vi "PutPlayerTrajectoryOnBoard.vi"(8 "error in (no error)":errorcluster, 9 "PlayerID":string="p1", 10 "PlayerTrajectory":T1[](array[typedef]), 11 "Board in":T4[][](array[typedef])) -> (0 "error out":errorcluster, 3 "Board out":T4[][](array[typedef]))   [LabVIEW 2015, in "TronviewPresentation.lvlib" / "BoardDisplay.lvclass"]
uses:
  BoardDisplay.lvclass
  TrajectoryBoardField.ctl
  TrajectoryFieldType.ctl
  TronVIEWBotAPI/MovementDirection.ctl
  PlayerTrajectory.ctl
  TronviewGame/Board/Position.ctl
  TronVIEWBotAPI/TronVIEWBotAPI.lvlib
  TronviewGame/Board/Board.lvclass
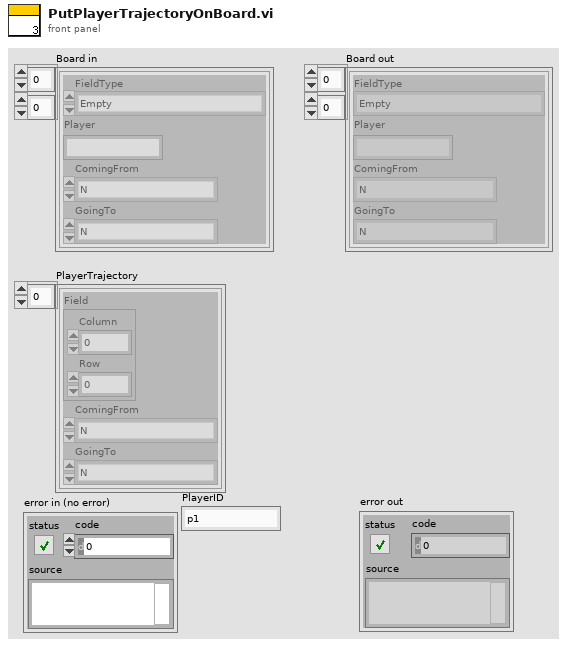
[diagram p1: front panel]
types:
  T1 = typedef "TronviewPresentation.lvlib/BoardDisplay.lvclass/PlayerTrajectory.ctl" = cluster{"Field":T2, "ComingFrom":T3, "GoingTo":T3}
  T2 = typedef "TronviewGame.lvlib/Board.lvclass/Position.ctl" = cluster{"Column":i32, "Row":i32}
  T3 = typedef "TronVIEWBotAPI.lvlib/MovementDirection.ctl" = enum16{"N", "S", "W", "E"}
  T4 = typedef "TronviewPresentation.lvlib/BoardDisplay.lvclass/TrajectoryBoardField.ctl" = cluster{"FieldType":T5, "Player":string, "ComingFrom":T3, "GoingTo":T3}
  T5 = typedef "TronviewPresentation.lvlib/BoardDisplay.lvclass/TrajectoryFieldType.ctl" = enum16{"Empty", "Initial", "PlayerWall", "PlayerPosition"}
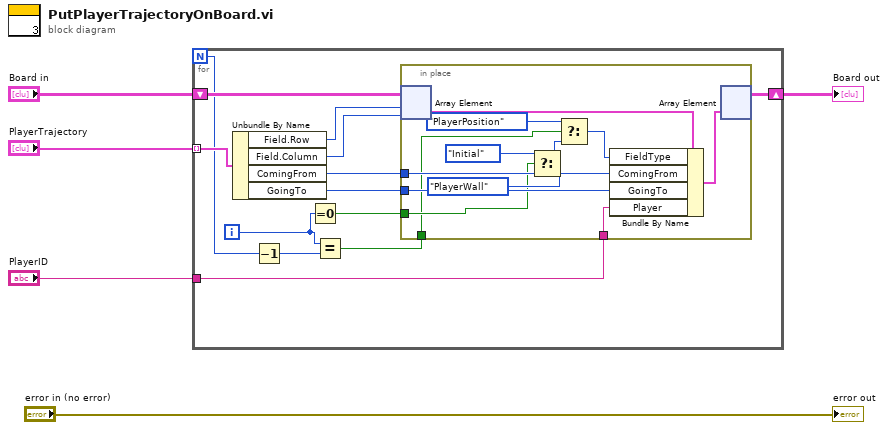
[diagram p0: block diagram]
diagram:
  n1 = for {
    N -> [w9]
    tunnel: "PlayerTrajectory" -> [w18] mode=indexing
    shift-right: [w12] -> w5
    shift-left: "Board in" -> [w17]
    tunnel: "PlayerID" -> [w6]
    i -> [w10]
    n2 = Unbundle By Name(w18) -> ("Field.Row"=w16:i32, "Field.Column"=w15:i32, "ComingFrom"=w14:T3, "GoingTo"=w13:T3)
    n3 = Decrement(x=w9) -> (x-1=w8:i32)
    n4 = Equal To 0?(x=w10) -> (x = 0?=w11:bool)
    n5 = Equal?(x=w10, y=w8) -> (x = y?=w7:bool)
    n6 = in-place {
      in-place-border: w14 -> [w28]
      in-place-border: w13 -> [w27]
      in-place-border: w11 -> [w24]
      in-place-border: w7 -> [w20]
      in-place-border: w6 -> [w19]
      n7 = in-place-array #1(w17, w16, w15) -> (w30:T4)
      n8 = Select(t=TrajectoryFieldType."Initial", s=w24, f=TrajectoryFieldType."PlayerWall" ("FieldType")) -> (s? t:f=w23:T5)
      n9 = Select(t=TrajectoryFieldType."PlayerPosition", s=w20, f=w23) -> (s? t:f=w22:T5)
      n10 = Bundle By Name(cluster=w30, "FieldType"=w22, "ComingFrom"=w28, "GoingTo"=w27, "Player"=w19) -> (w29:T4)
      n11 = in-place-array #1(w29) -> (w12:T4[][])  [unwired: 2 out]
    }
  }
  "Board out" <- w5
  "error out" <- "error in (no error)"
